vi "ParseLeidenComputerNames.vi"() -> ()   [LabVIEW 2013]
panel:
  out "is windysea?":bool
  out "Type":enum32{"CF", "Wet"}(ring)
  out "is gallowspole?":bool
  out "is custardpie?":bool
  in  "computer name":string="custardpie"
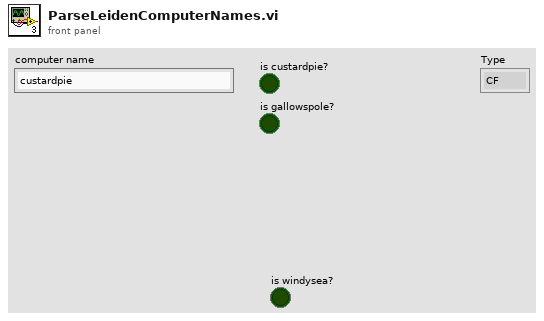
[diagram p1: front panel]
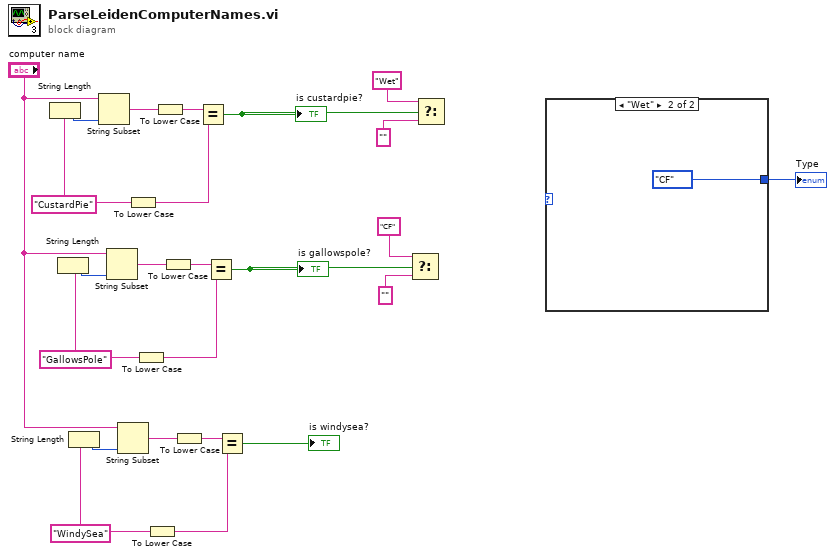
[diagram p0: block diagram]
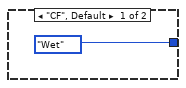
[diagram p2: hidden frame]
diagram:
  w12 = "WindySea"
  w16 = "GallowsPole"
  w23 = "CustardPie"
  n1 = String Length(string=w23) -> (length=w22:i32)
  n2 = String Length(string=w16) -> (length=w17:i32)
  n3 = String Length(string=w12) -> (length=w11:i32)
  n4 = String Subset(string="computer name", length (rest)=w22) -> (substring=w24:string)  [unwired: 1 in]
  n5 = String Subset(string="computer name", length (rest)=w17) -> (substring=w15:string)  [unwired: 1 in]
  n6 = String Subset(string="computer name", length (rest)=w11) -> (substring=w13:string)  [unwired: 1 in]
  n7 = To Lower Case(string=w23) -> (all lower case string=w21:string)
  n8 = To Lower Case(string=w16) -> (all lower case string=w18:string)
  n9 = To Lower Case(string=w12) -> (all lower case string=w10:string)
  n10 = To Lower Case(string=w24) -> (all lower case string=w20:string)
  n11 = To Lower Case(string=w15) -> (all lower case string=w19:string)
  n12 = To Lower Case(string=w13) -> (all lower case string=w9:string)
  n13 = Equal?(x=w20, y=w21) -> (x = y?=w6:bool)
  "is custardpie?" <- w6
  n14 = Equal?(x=w19, y=w18) -> (x = y?=w4:bool)
  "is gallowspole?" <- w4
  n15 = Equal?(x=w9, y=w10) -> (x = y?=→"is windysea?":bool)
  n16 = Select(t="CF", s=w4, f="") -> ()  [unwired: 1 out]
  n17 = Select(t="Wet", s=w6, f="") -> ()  [unwired: 1 out]
  n18 = case shown="\"Wet\"" {
    selector: _ -> [_ _]
    tunnel: [enum32{"CF", "Wet"}."Wet" ("Type") enum32{"CF", "Wet"}."CF" ("Type")] -> w7
    frame "CF", Default {
    }
    frame "Wet" {
    }
  }
  "Type" <- w7
